vi "ThrottleAngleToArea.vi"(1 "Throttle Angle":sgl caption="deg") -> (0 "Throttle Area":sgl)   [LabVIEW 2016, in "NI-PCG Vehicle Model.lvlib"]
uses:
  NI-PCG Vehicle Model.lvlib
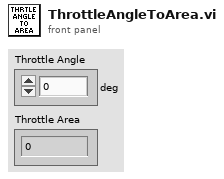
[diagram p1: front panel]
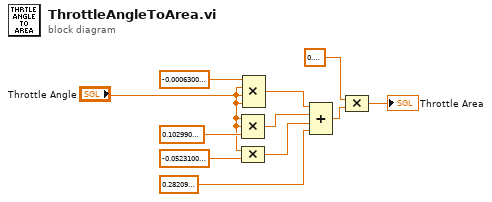
[diagram p0: block diagram]
diagram:
  n1 = Compound Arithmetic op=MULTIPLY("Throttle Angle", "Throttle Angle", sgl 0.10299 ("value")) -> (w7:sgl)
  n2 = Compound Arithmetic op=MULTIPLY("Throttle Angle", sgl -0.05231 ("value")) -> (w6:sgl)
  n3 = Compound Arithmetic op=MULTIPLY(sgl -0.00063 ("value"), "Throttle Angle", "Throttle Angle", "Throttle Angle") -> (w8:sgl)
  n4 = Compound Arithmetic op=ADD(w8, w7, w6, sgl 0.2821 ("value")) -> (w4:sgl)
  n5 = Compound Arithmetic op=MULTIPLY(sgl 0.6 ("value"), w4) -> (→"Throttle Area":sgl)
